vi "set phase sampling info duty cycle.vi"(8 "error in (no error)":errorcluster, 11 "Waveform in":refnum<class "Waveform.lvclass">) -> (0 "error out":errorcluster, 3 "Waveform out":refnum<class "Waveform.lvclass">)   [LabVIEW 2012, in "Waveform.lvclass"]
uses:
  Waveform.lvclass
  Waveform.lvclass/Waveform.ctl
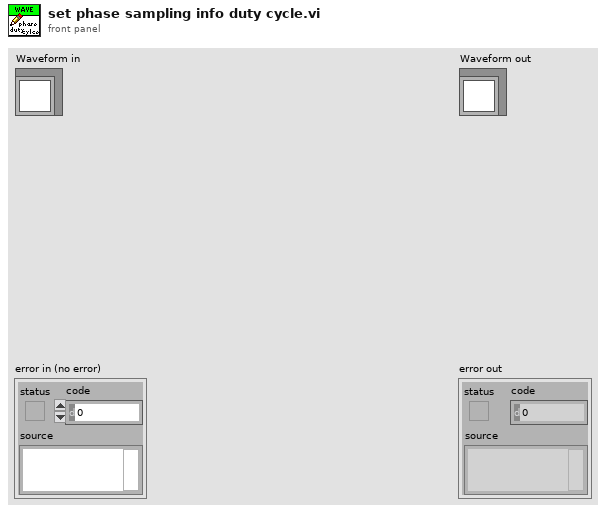
[diagram p1: front panel]
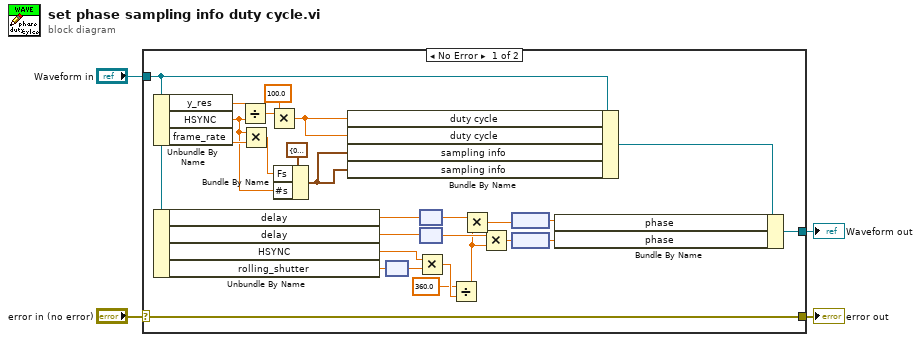
[diagram p0: block diagram]
diagram:
  n1 = case shown="No Error" "error in (no error)" {
    selector: "error in (no error)" -> [w31 w33]
    tunnel: [w31 w33] -> w3
    tunnel: [w12 w32] -> w1
    tunnel: "Waveform in" -> [w21 w32]
    frame No Error {
      n2 = Unbundle By Name(w21) -> ("y_res"=w30:dbl, "HSYNC"=w23:dbl, "frame_rate"=w26:dbl)
      n3 = Unbundle By Name(w21) -> ("delay"=w20:dbl[unit], "delay"=w19:dbl[unit], "HSYNC"=w9:dbl, "rolling_shutter"=w11:dbl[unit])
      n4 = Divide(x=w30, y=w23) -> (x/y=w29:dbl)
      n5 = Multiply(x=w23, y=w26) -> (x*y=w24:dbl)
      n6 = Multiply(x=w29, y=100.0) -> (x*y=w27:dbl)
      n7 = Bundle By Name(cluster=cluster{"Fs":dbl, "#s":dbl} {"Fs"=0.0, "#s"=0.0} ("settings.Pockels Cell.sampling info"), "Fs"=w24, "#s"=w23) -> (w22:cluster{"Fs":dbl, "#s":dbl})
      n8 = Bundle By Name(cluster=w21, "duty cycle"=w27, "duty cycle"=w27, "sampling info"=w22, "sampling info"=w22) -> (w14:refnum<class "Waveform.lvclass">)
      n9 = node(w11) -> (w10:dbl)
      n10 = Multiply(x=w9, y=w10) -> (x*y=w8:dbl)
      n11 = node(w20) -> (w18:dbl)
      n12 = node(w19) -> (w6:dbl)
      n13 = Divide(x=360.0, y=w8) -> (x/y=w5:dbl)
      n14 = Multiply(x=w18, y=w5) -> (x*y=w17:dbl)
      n15 = Multiply(x=w6, y=w5) -> (x*y=w16:dbl)
      n16 = node(w17) -> (w15:dbl[unit])
      n17 = node(w16) -> (w13:dbl[unit])
      n18 = Bundle By Name(cluster=w14, "phase"=w15, "phase"=w13) -> (w12:refnum<class "Waveform.lvclass">)
    }
    frame Error {
    }
  }
  "error out" <- w3
  "Waveform out" <- w1
